vi "Test Return Aggregated Result for Error Parametrized Case.vi"(11 "Test Case In":refnum<class "Parameterized Test Case Test.lvclass">) -> (0 "error out":errorcluster, 3 "Test Case Out":refnum<class "Parameterized Test Case Test.lvclass">)   [LabVIEW 2020, in "Parameterized Test Case Test.lvclass"]
uses:
  Parameterized Test Case Test.lvclass
  C:/Program Files/National Instruments/LabVIEW 2024/vi.lib/Astemes/LUnit/Test Case.lvclass
  <vilib>/Astemes/LUnit/Test Case.lvclass/Test Case.ctl
  41b79fda-963b-489b-a42a-568db35b7394.vi
  <vilib>/Astemes/LUnit/Core/LUnit Test Case/Private/Append Pass Result.vi
  <vilib>/Astemes/LUnit/Core/LUnit Test Case/Private/Append Fail Result.vi
  41b79fda-963b-489b-a42a-568db35b7394.vi/9c5d11cd-9439-4240-a1ee-d9baace9c924.vi
  <vilib>/Astemes/LUnit/Core/LUnit Test Case/Private/Run In UI.vi
  <vilib>/Utility/error.llb/Clear Errors.vi
  source/Parameterized Test Case/Parameterized Test Case.lvclass
  <vilib>/Astemes/LUnit/Test Suite.lvclass
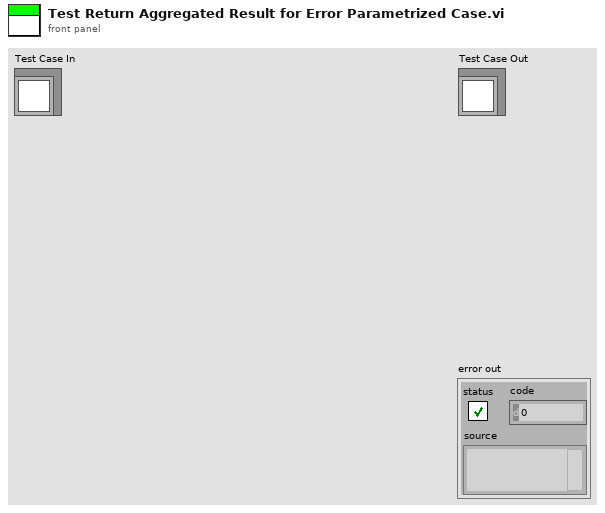
[diagram p1: front panel]
types:
  T1 = enum16{"", "Passed", "Failed", "Error", "Skipped", "Setup Error", "Broken", "Teardown Error"}
  T2 = cluster{"Name":string, "Description":string, "Status":enum16{"", "Passed", "Failed", "Error", "Skipped", "Setup Error", "Broken", "Teardown Error"}, "Result Type":enum16{"Test Case", "Test Suite", "Test Run", "Pass", "Fail", "Skip", "Pass if", "Fail if", "Pass if Error", "Fail if Error", "Pass if Equal", "Fail if Equal"}, "Execution Time":dbl, "Data":cluster{"Expected":variant, "Actual":variant, "Delta":variant}}[]
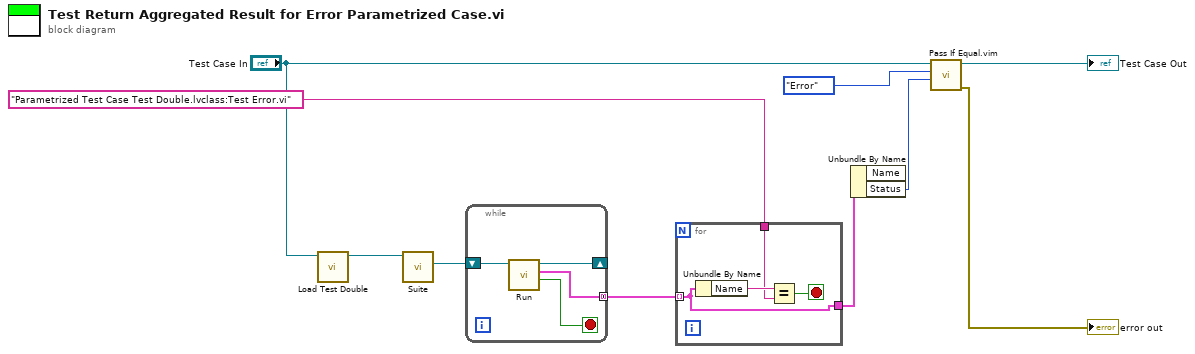
[diagram p0: block diagram]
diagram:
  n1 = call "Load Test Double.vi"("Parameterized Test Case Test in"="Test Case In") -> ("Parameterized Test Case out"=w1:refnum<class "Parameterized Test Case.lvclass">)  [unwired: 9 in, 1 out]
  n2 = call-dynamic "Suite.vi"("Parameterized Test Case In"=w1) -> ("LUnit Test Suite Out"=w8:refnum<class "Test Suite.lvclass">)  [unwired: 8 in, 2 out]
  n3 = while {
    tunnel: [w14] -> w7 mode=concatenating
    shift-right: [w12] -> _
    shift-left: w8 -> [w13]
    stop <- w11 stop-if-true
    n4 = call-dynamic "Run.vi"("LUnit Test Suite In"=w13) -> ("Done?"=w11:bool, "Results"=w14:T2, "LUnit Test Suite In 2"=w12:refnum<class "Test Suite.lvclass">)  [unwired: 7 in, 1 out]
  }
  n5 = for {
    tunnel: w7 -> [w15] mode=indexing
    tunnel: "Parametrized Test Case Test Double.lvclass:Test Error.vi" ("String") -> [w17]
    tunnel: [w15] -> w3
    stop <- w16 stop-if-true
    n6 = Unbundle By Name(w15) -> ("Name"=w18:string)
    n7 = Equal?(x=w18, y=w17) -> (x = y?=w16:bool)
  }
  n8 = Unbundle By Name(w3) -> ("Status"=w4:T1)  [unwired: 1 out]
  n9 = call "Pass If Equal.vim"("Actual"=w4, "Expected"=T1."Error" ("Status"), "LUnit Test Case In"="Test Case In") -> ("error out"=→"error out":errorcluster, "LUnit Test Case Out"=→"Test Case Out":refnum<class "Parameterized Test Case Test.lvclass">)  [unwired: 7 in]
